vi "DiffWheel_Normalize.vi"(6 "Max Speed":dbl, 9 "Right Wheel Demand":dbl, 11 "Left Wheel Demand":dbl) -> (1 "Normalized Right Wheel Demand":dbl, 3 "Normalized Left Wheel Demand":dbl)   [LabVIEW 2019, in "Trajectory_Library.lvlib"]
doc: "Normalizes the wheel speeds using some max attainable speed. Sometimes, after inverse kinematics, the requested speed from a/several modules may be above the max attainable speed for the driving motor on that module. To fix this issue, one can \"normalize\" all the wheel speeds to make sure that all requested module speeds are below the absolute threshold, while maintaining the ratio of speeds between modules.\n\nParameters:\n - Left Wheel Demand - Desired left wheel speed demand.\n - Right Wheel Demand - Desired right wheel speed demand.\n - Max Speed - The absolute max speed that a wheel can reach.\n\nReturns:\n - Normalized Left Wheel Demand\n - Normalized Right Wheel Demand"
uses:
  Trajectory_Library.lvlib
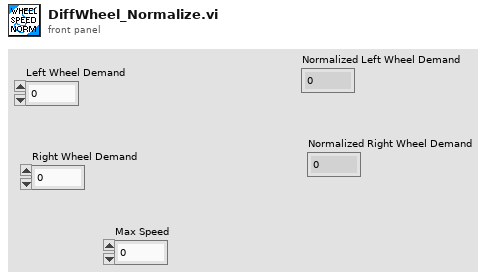
[diagram p1: front panel]
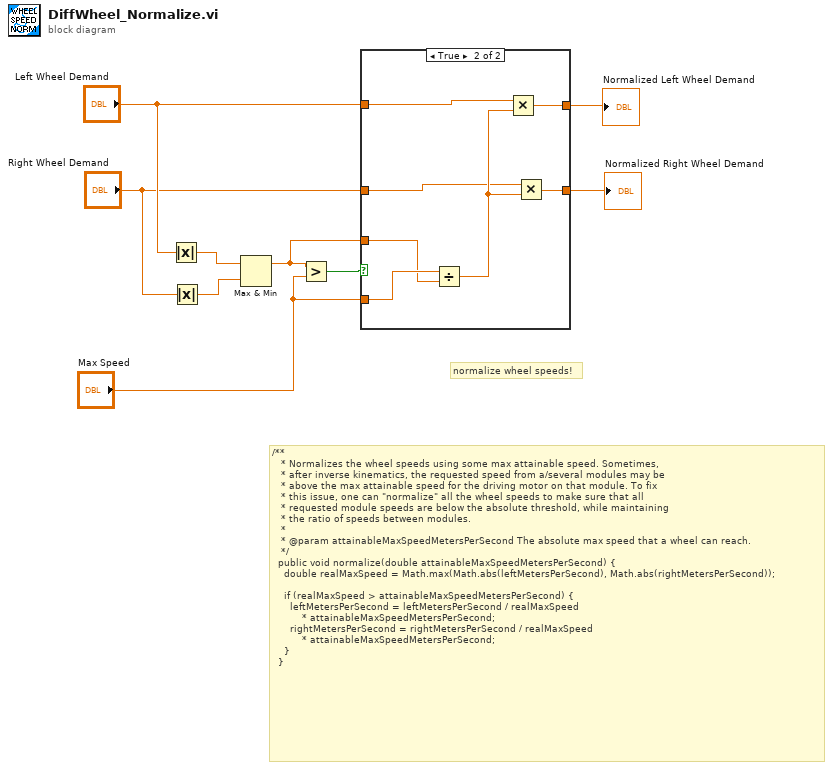
[diagram p0: block diagram]
diagram:
  # "/**\n   * Normalizes the wheel speeds using some max attainable speed. Sometimes,\n   * after inverse kinematics, the requested speed from a/several modules may be\n   * above the max attainable speed for the driving motor on that module. To fix\n   * this issue, one can \"normalize\" all the wheel speeds to make sure that all\n   * requested module speeds are below the absolute threshold, while maintaining\n   * the ratio of speeds between modules.\n   *\n   * @param attainableMaxSpeedMetersPerSecond The absolute max speed that a wheel can reach.\n   */\n  public void normalize(double attainableMaxSpeedMetersPerSecond) {\n    double realMaxSpeed = Math.max(Math.abs(leftMetersPerSecond), Math.abs(rightMetersPerSecond));\n\n    if (realMaxSpeed > attainableMaxSpeedMetersPerSecond) {\n      leftMetersPerSecond = leftMetersPerSecond / realMaxSpeed\n          * attainableMaxSpeedMetersPerSecond;\n      rightMetersPerSecond = rightMetersPerSecond / realMaxSpeed\n          * attainableMaxSpeedMetersPerSecond;\n    }\n  }"
  # "normalize wheel speeds!"
  n1 = Absolute Value(x="Left Wheel Demand") -> (abs(x)=w9:dbl)
  n2 = Absolute Value(x="Right Wheel Demand") -> (abs(x)=w8:dbl)
  n3 = Max & Min(x=w9, y=w8) -> (max(x,y)=w2:dbl)  [unwired: 1 out]
  n4 = Greater?(x=w2, y="Max Speed") -> (0:w1:bool)
  n5 = case shown="True" w1 {
    tunnel: [w11 w14] -> w5
    tunnel: "Left Wheel Demand" -> [w11 w13]
    tunnel: "Right Wheel Demand" -> [w10 w12]
    tunnel: [w10 w15] -> w4
    tunnel: "Max Speed" -> [_ w18]
    tunnel: w2 -> [_ w17]
    frame False {
    }
    frame True {
      n6 = Divide(x=w18, y=w17) -> (x/y=w16:dbl)
      n7 = Multiply(x=w13, y=w16) -> (x*y=w14:dbl)
      n8 = Multiply(x=w12, y=w16) -> (x*y=w15:dbl)
    }
  }
  "Normalized Left Wheel Demand" <- w5
  "Normalized Right Wheel Demand" <- w4
